vi "Heise Barometric Pressure 901A Parse Data Stream.vi"(8 "Error In":errorcluster, 10 "Data Stream":string) -> (0 "Error Out":errorcluster, 2 "Barometric Pressure (in. Hg) String":string, 3 "Barometric Pressure (in. Hg)":dbl)   [LabVIEW 2018]
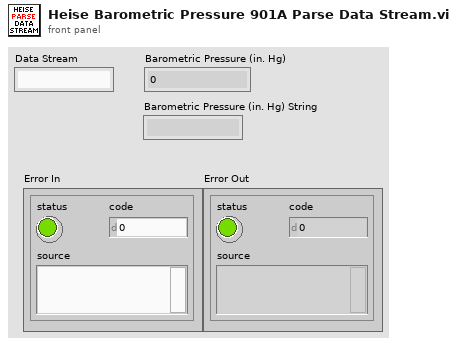
[diagram p1: front panel]
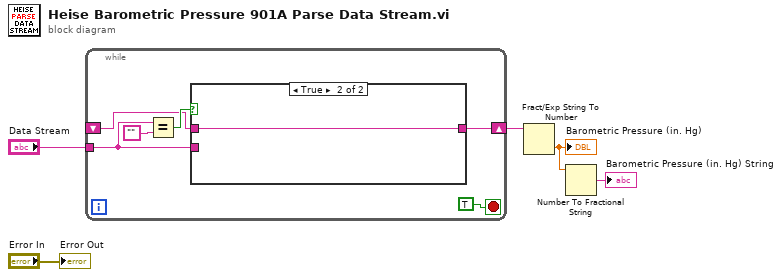
[diagram p0: block diagram]
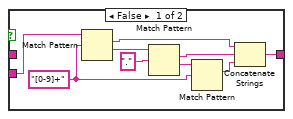
[diagram p2: hidden frame]
diagram:
  n1 = while {
    shift-right: [w11] -> w5
    shift-left: _ -> [w6]
    tunnel: "Data Stream" -> [w7]
    stop <- TRUE stop-if-true
    n2 = Equal?(x=w7, y="") -> (x = y?=w8:bool)
    n3 = case shown="True" w8 {
      tunnel: [w19 w21] -> w11
      tunnel: w7 -> [w12 _]
      tunnel: w6 -> [_ w21]
      frame False {
        w20 = "[0-9]+" ("regular expression")
        n4 = Match Pattern(string=w12, regular expression=w20) -> (match substring=w16:string, after substring=w13:string)  [unwired: 1 in, 2 out]
        n5 = Match Pattern(string=w13, regular expression=".") -> (match substring=w17:string, after substring=w15:string)  [unwired: 1 in, 2 out]
        n6 = Match Pattern(string=w15, regular expression=w20) -> (match substring=w18:string)  [unwired: 1 in, 3 out]
        n7 = Concatenate Strings(w16, w17, w18) -> (w19:string)
      }
      frame True {
      }
    }
  }
  n8 = Fract/Exp String To Number(string=w5) -> (number=w2:dbl)  [unwired: 3 in, 1 out]
  "Barometric Pressure (in. Hg)" <- w2
  n9 = Number To Fractional String(number=w2) -> (F-format string=→"Barometric Pressure (in. Hg) String":string)  [unwired: 3 in]
  "Error Out" <- "Error In"
